vi "GDSIconEditor_FindPrefixInfo.vi"(0 "_VIPath":path, 9 "Folder":path, 11 "error in (no error)":errorcluster) -> (4 "FolderFiles":path[](array[path]), 6 "Prefix":string, 8 "Separator":string, 10 "name":string, 14 "FilePreFix+Separtor":string, 15 "error out":errorcluster)   [LabVIEW 2016]
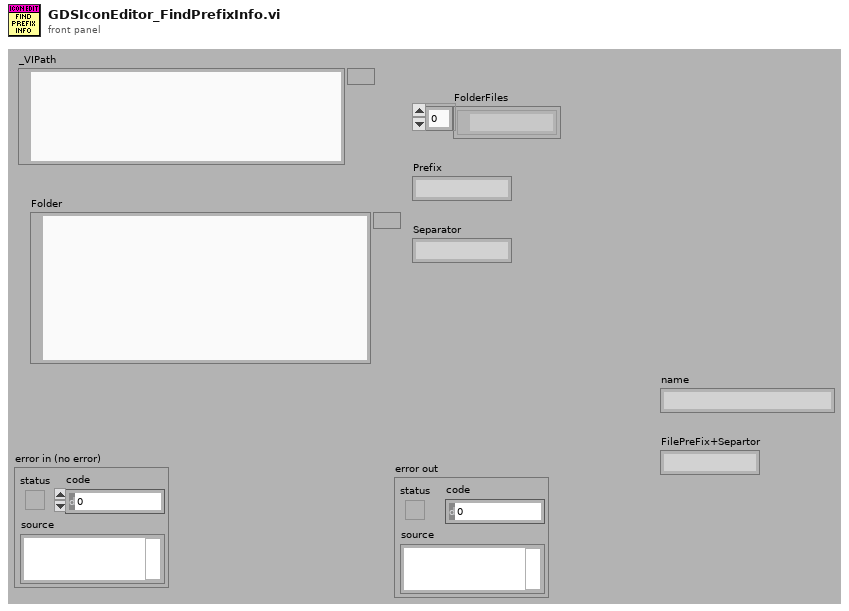
[diagram p1: front panel]
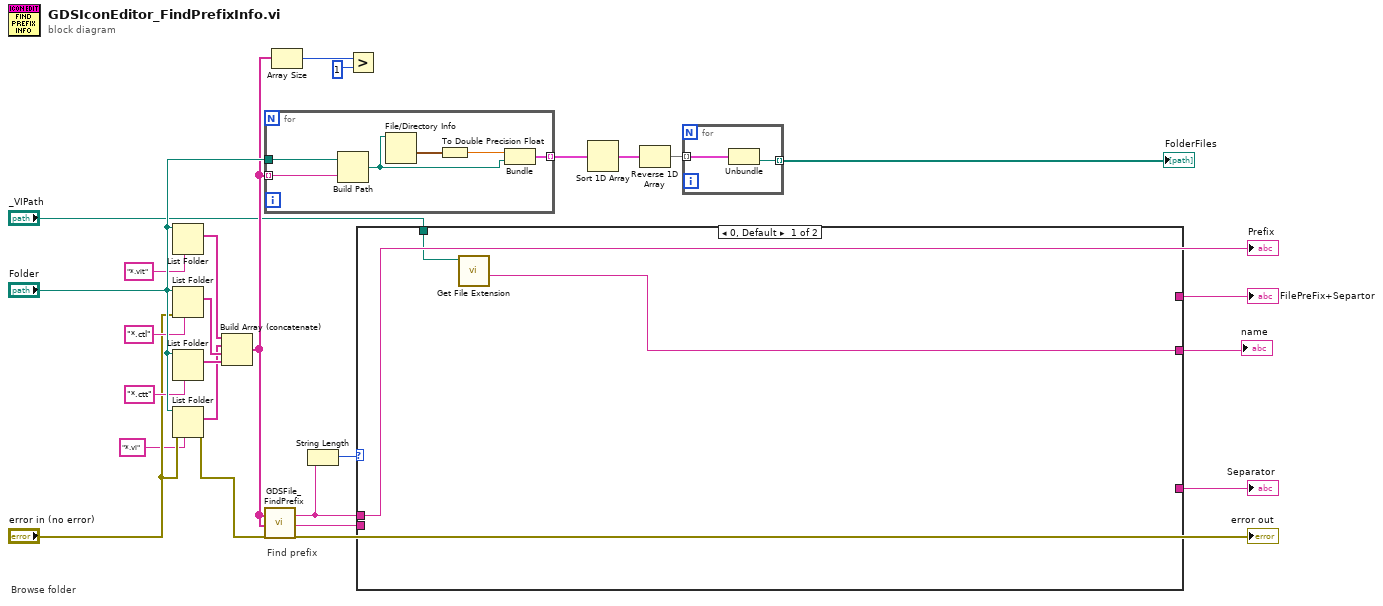
[diagram p0: block diagram]
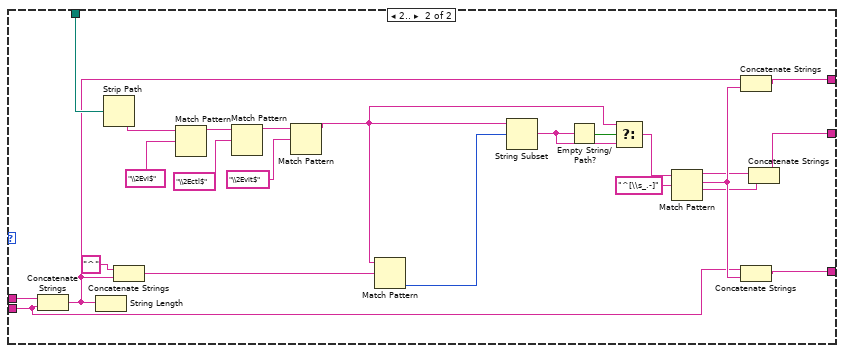
[diagram p2: hidden frame]
diagram:
  # "Browse folder"
  # "Find prefix"
  n1 = List Folder(path="Folder", pattern="*.vit") -> (filenames=w21:string[])  [unwired: 2 in, 3 out]
  n2 = List Folder(path="Folder", pattern="*.ctl", error in="error in (no error)") -> (filenames=w22:string[])  [unwired: 1 in, 3 out]
  n3 = List Folder(path="Folder", pattern="*.ctt") -> (filenames=w23:string[])  [unwired: 2 in, 3 out]
  n4 = List Folder(path="Folder", pattern="*.vi", error in="error in (no error)") -> (filenames=w12:string[], error out=w11:errorcluster)  [unwired: 1 in, 2 out]
  n5 = Build Array (concatenate)(w21, w12, w22, w23) -> (w16:string[])
  n6 = for {
    tunnel: "Folder" -> [w32]
    tunnel: w16 -> [w31] mode=indexing
    tunnel: [w29] -> w13 mode=indexing
    n7 = Build Path(base path=w32, name or relative path=w31) -> (appended path=w30:path)
    n8 = File/Directory Info(path=w30) -> (last mod=w28:timestamp)  [unwired: 1 in, 6 out]
    n9 = To Double Precision Float(number=w28) -> (double precision float=w27:dbl)
    n10 = Bundle(w27, "appended path"=w30) -> (w29:cluster{dbl, "appended path":path})  [unwired: 1 in]
  }
  n11 = call <resource>:"GDSFile_FindPrefix.vi"("Filenames as references"=w16, "Filenames to search"=w16, "error in (no error)"=w11) -> ("Prefix"=w2:string, "Separator"=w5:string, "error out"=→"error out":errorcluster)  [unwired: 14 in]
  "Prefix" <- w2
  n12 = Array Size(array=w16) -> (size(s)=w8:i32)
  n13 = String Length(string=w2) -> (length=w1:i32)
  n14 = Greater?(x=w8, y=1) -> ()  [unwired: 1 out]
  n15 = case shown="0, Default" w1 {
    tunnel: "_VIPath" -> [w34 w58]
    tunnel: [_ w43] -> w6
    tunnel: w5 -> [_ w41]
    tunnel: [_ w40] -> w4
    tunnel: [w33 w36] -> w3
    tunnel: w2 -> [_ w35]
    frame 0, Default {
      n16 = call <vilib>:"Get File Extension.vi"("file"=w34) -> ("filename without extension"=w33:string)  [unwired: 6 in, 4 out]
    }
    frame 2.. {
      n17 = Concatenate Strings(w35, w41) -> (w44:string)
      n18 = String Length(string=w44) -> ()  [unwired: 1 out]
      n19 = Strip Path(path=w58) -> (name=w50:string)  [unwired: 1 out]
      n20 = Concatenate Strings("^", w44) -> (w51:string)
      n21 = Match Pattern(string=w50, regular expression="\\2Evi$") -> (before substring=w55:string)  [unwired: 1 in, 3 out]
      n22 = Match Pattern(string=w55, regular expression="\\2Ectl$") -> (before substring=w54:string)  [unwired: 1 in, 3 out]
      n23 = Match Pattern(string=w54, regular expression="\\2Evit$") -> (before substring=w48:string)  [unwired: 1 in, 3 out]
      n24 = Match Pattern(string=w48, regular expression=w51) -> (offset past match=w46:i32)  [unwired: 1 in, 3 out]
      n25 = String Subset(string=w48, offset (0)=w46) -> (substring=w47:string)  [unwired: 1 in]
      n26 = Empty String/Path?(string/path=w47) -> (empty?=w49:bool)
      n27 = Select(t=w48, s=w49, f=w47) -> (s? t:f=w37:string)
      n28 = Match Pattern(string=w37, regular expression="^[\\s_.-]") -> (before substring=w39:string, match substring=w42:string, after substring=w38:string)  [unwired: 1 in, 1 out]
      n29 = Concatenate Strings(w44, w42) -> (w43:string)
      n30 = Concatenate Strings(w41, w42) -> (w40:string)
      n31 = Concatenate Strings(w39, w38) -> (w36:string)
    }
  }
  "FilePreFix+Separtor" <- w6
  "name" <- w3
  "Separator" <- w4
  n32 = Sort 1D Array(array=w13) -> (sorted array=w14:cluster{dbl, "appended path":path}[])
  n33 = Reverse 1D Array(array=w14) -> (reversed array=w25:cluster{dbl, "appended path":path}[])
  n34 = for {
    tunnel: w25 -> [w60] mode=indexing
    tunnel: [w59] -> w26 mode=indexing
    n35 = Unbundle(w60) -> ("appended path"=w59:path)  [unwired: 1 out]
  }
  "FolderFiles" <- w26
